vi "FlatToRichcif_channelcore_Channel.vi"(5 "OutputClusterType":T1, 11 "InputCluster":T3) -> (3 "OutputCluster":T1)   [LabVIEW 2021, in "CIFCoreChannel_client.lvlib"]
uses:
  CIFCoreChannel_client.lvlib
  cif_channelcore_Channel_Flat.ctl
  cif_channelcore_Direction.ctl
  cif_channelcore_Channel.ctl
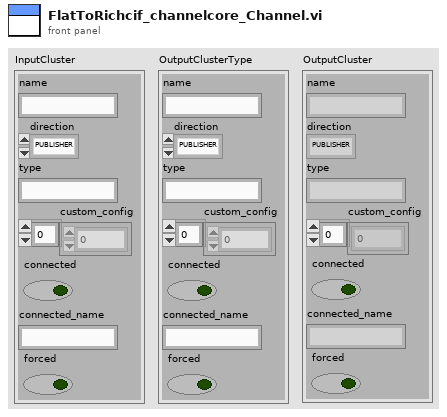
[diagram p1: front panel]
types:
  T1 = typedef "CIFCoreChannel_client.lvlib/cif_channelcore_Channel.ctl" = cluster{"name":string, "direction":T2, "type":string, "custom_config":u8[], "connected":bool, "connected_name":string, "forced":bool}
  T2 = typedef "CIFCoreChannel_client.lvlib/cif_channelcore_Direction.ctl" = enum32{"PUBLISHER", "SUBSCRIBER"}
  T3 = typedef "CIFCoreChannel_client.lvlib/cif_channelcore_Channel_Flat.ctl" = cluster{"name":string, "direction":T2, "type":string, "custom_config":u8[], "connected":bool, "connected_name":string, "forced":bool}
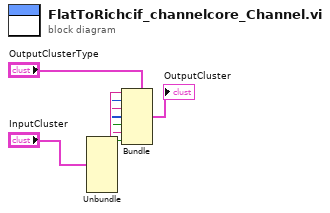
[diagram p0: block diagram]
diagram:
  n1 = Unbundle "Unbundle"("InputCluster") -> ("name"=w7:string, "direction"=w6:T2, "type"=w5:string, "custom_config"=w4:u8[], "connected"=w3:bool, "connected_name"=w2:string, "forced"=w1:bool)
  n2 = Bundle "Bundle"(cluster="OutputClusterType", "name"=w7, "direction"=w6, "type"=w5, "custom_config"=w4, "connected"=w3, "connected_name"=w2, "forced"=w1) -> (→"OutputCluster":T1)
